vi "UI-RT Communication.vi"(8 "error in (no error)":errorcluster) -> (0 "error out":errorcluster)   [LabVIEW 2016]
uses:
  Controls/Message Structure.ctl
  Controls/Operational Modes.ctl
  Controls/Shutter Manual.ctl
  Controls/Flip Mirror Manual.ctl
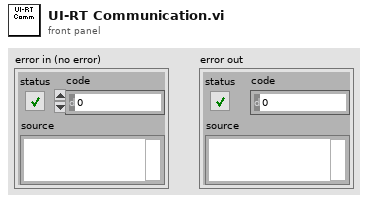
[diagram p1: front panel]
types:
  T1 = typedef "Message Structure.ctl" = cluster{"Data":variant, "Cmd":string}
  T2 = typedef "Operational Modes.ctl" = enum16{"Sci", "Sci-LFC", "Solar", "Solar-LFC", "LFC", "LFC-Sim", "LFC-Both", "ThAr", "ThAr-LFC", "Flat", "ExtFlat", "ExtFlat-Sim", "ExtFlat-Both", "Qtz", "ExtQtz", "ExtQtz-Sim", "ExtQtz-Both", "Dark", "Manual", "Off"}
  T3 = typedef "Shutter Manual.ctl" = cluster{"Science":bool, "Solar":bool, "Ext Flat":bool, "Sim LFC":bool, "Sim Flat":bool}
  T4 = typedef "Flip Mirror Manual.ctl" = cluster{"ExtFlat":bool, "Solar":bool, "ThAr":bool}
  T5 = typedef "Shutters.ctl" = cluster{"Science":T6, "LFCSim":T6, "ExtendFlat":T6, "SimFlat":T6, "Solar":T6}
  T6 = typedef "Shutter Data.ctl" = cluster{"Status":bool, "State":T7, "Time Stamps":cluster{"Open":timestamp, "Close":timestamp}, "Exposure Time":dbl}
  T7 = typedef "Shutter States.ctl" = enum16{"Open", "Close", "Wait", "Off", "Arm", "Idle"}
  T8 = typedef "Flip Mirrors.ctl" = cluster{"ExtFlat":T9, "ThAr":T9, "Solar":T9}
  T9 = typedef "Mirror Data.ctl" = cluster{"Status":bool, "Time Stamp":timestamp}
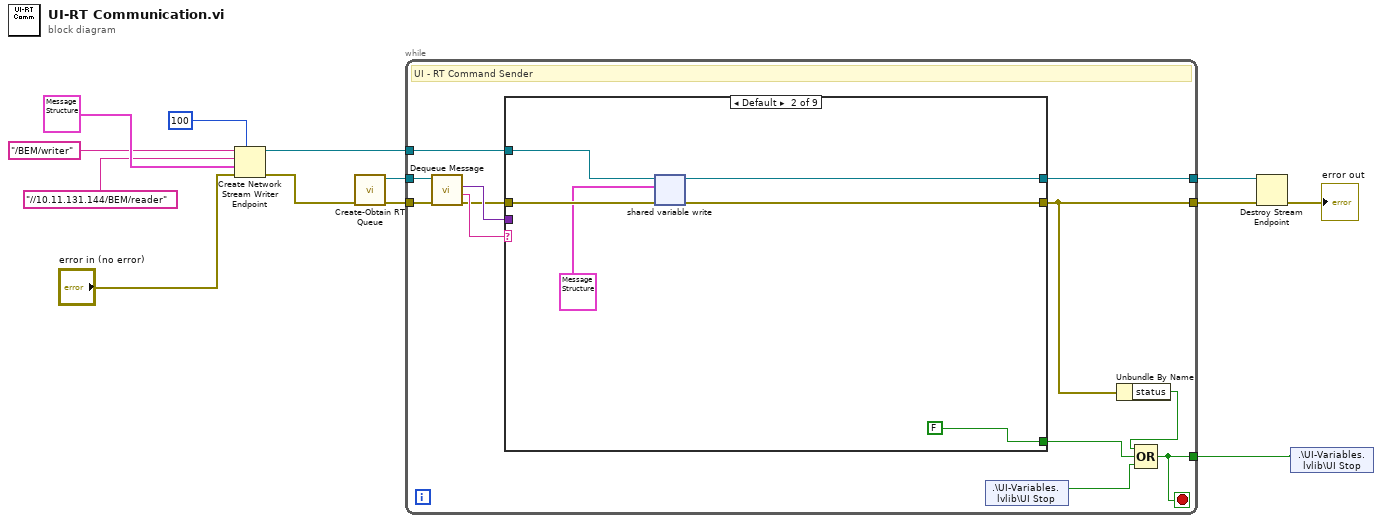
[diagram p0: block diagram]
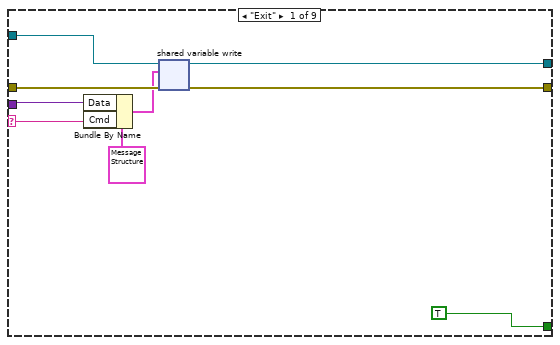
[diagram p2: hidden frame]
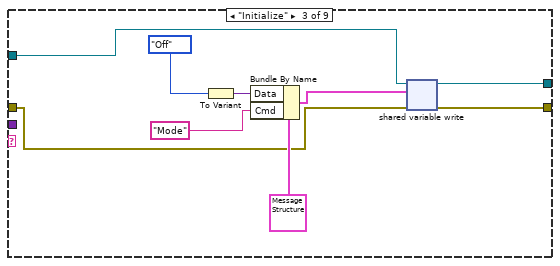
[diagram p3: hidden frame]
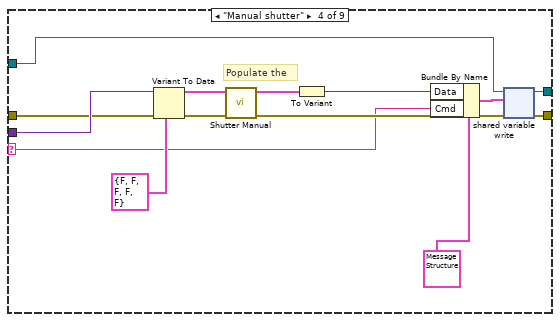
[diagram p4: hidden frame]
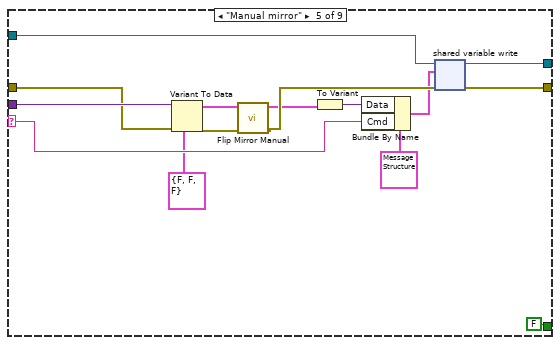
[diagram p5: hidden frame]
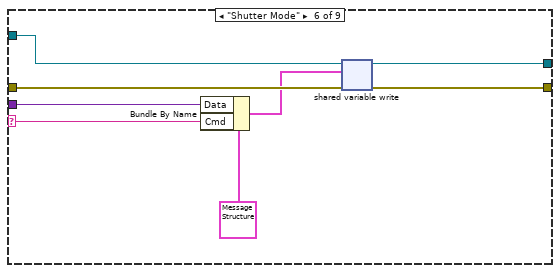
[diagram p6: hidden frame]
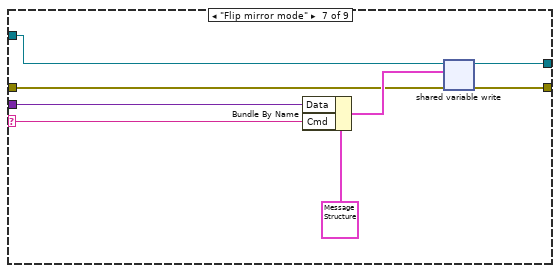
[diagram p7: hidden frame]
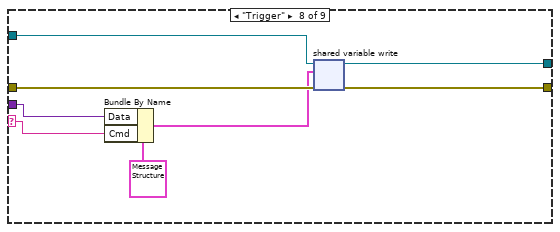
[diagram p8: hidden frame]
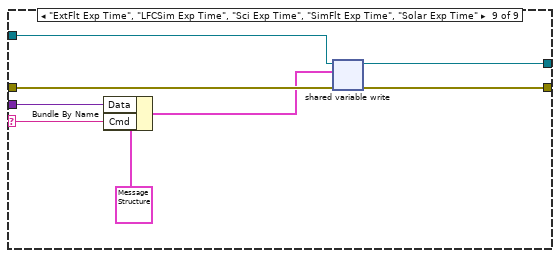
[diagram p9: hidden frame]
diagram:
  n1 = Create Network Stream Writer Endpoint(7:100 ("writer buffer size"), 8:"error in (no error)", 9:T1 {"Data"=variant, "Cmd"=""}, 10:"//10.11.131.144/BEM/reader", 11:"/BEM/writer" ("writer name")) -> (0:w2:errorcluster, 3:w10:refnum<k21>)  [unwired: 2 in]
  n2 = call "Create-Obtain RT Queue.vi"("error in (no error)"=w2) -> ("error out"=w1:errorcluster, "Queue out"=w3:refnum<queue>)  [unwired: 8 in, 1 out]
  n3 = while {
    tunnel: w3 -> [w17]
    tunnel: w10 -> [w25]
    tunnel: [w19] -> w4
    tunnel: w1 -> [w18]
    tunnel: [w22] -> w6
    tunnel: [w21] -> w7
    stop <- w21 stop-if-true
    # "UI - RT Command Sender"
    n4 = call "Dequeue Message.vi"("error in (no error)"=w18, "Queue in"=w17) -> ("error out"=w14:errorcluster, "Cmd"=w16:string, "Data"=w15:variant)  [unwired: 6 in, 1 out]
    n5 = case shown="Default" w16 {
      selector: w16 -> [w27 _ _ w52 w77 w81 w87 w96 w105]
      tunnel: [TRUE FALSE _ _ FALSE _ _ _ _] -> w24
      tunnel: w15 -> [w28 _ _ w63 w76 w82 w88 w97 w104]
      tunnel: w14 -> [w33 w39 w41 w62 w66 w84 w90 w99 w108]
      tunnel: w25 -> [w32 w38 w47 w57 w74 w80 w89 w102 w107]
      tunnel: [w31 w37 w48 w59 w73 w85 w92 w100 w109] -> w19
      tunnel: [w30 w36 w49 w58 w75 w86 w91 w101 w110] -> w22
      frame "Exit" {
        n6 = Bundle By Name(cluster=T1 {"Data"=variant, "Cmd"=""} ("Message"), "Data"=w28, "Cmd"=w27) -> (w26:T1)
        n7 = shared-variable-write(w32, w33, w26) -> (w30:refnum<k21>, w31:errorcluster)  [unwired: 1 in, 1 out]
      }
      frame Default {
        n8 = shared-variable-write(w38, w39, T1 {"Data"=variant, "Cmd"=""} ("Message")) -> (w36:refnum<k21>, w37:errorcluster)  [unwired: 1 in, 1 out]
      }
      frame "Initialize" {
        n9 = To Variant(anything=Operational_Modes."Off" ("EXPRES Mode 2")) -> (Variant=w46:variant)
        n10 = Bundle By Name(cluster=T1 {"Data"=variant, "Cmd"=""} ("Message"), "Data"=w46, "Cmd"="Mode") -> (w43:T1)
        n11 = shared-variable-write(w47, w41, w43) -> (w49:refnum<k21>, w48:errorcluster)  [unwired: 1 in, 1 out]
      }
      frame "Manual shutter" {
        # "Populate the"
        n12 = Variant To Data(error in=w62, type=T3 {"Science"=FALSE, "Solar"=FALSE, "Ext Flat"=FALSE, "Sim LFC"=FALSE, "Sim Flat"=FALSE} ("Manual Shutter 2"), Variant=w63) -> (data=w60:T3, error out=w55:errorcluster)
        n13 = call "Shutter Manual.vi"("Error In"=w55, "Manual Shutter in"=w60) -> ("Error Out"=w54:errorcluster, "Shutters out"=w53:T5)  [unwired: 8 in]
        n14 = To Variant(anything=w53) -> (Variant=w56:variant)
        n15 = Bundle By Name(cluster=T1 {"Data"=variant, "Cmd"=""} ("Message"), "Data"=w56, "Cmd"=w52) -> (w50:T1)
        n16 = shared-variable-write(w57, w54, w50) -> (w58:refnum<k21>, w59:errorcluster)  [unwired: 1 in, 1 out]
      }
      frame "Manual mirror" {
        n17 = Variant To Data(error in=w66, type=T4 {"ExtFlat"=FALSE, "Solar"=FALSE, "ThAr"=FALSE} ("Manual Mirror"), Variant=w76) -> (data=w68:T4, error out=w71:errorcluster)
        n18 = call "Flip Mirror Manual.vi"("error in (no error)"=w71, "Manual Mirror"=w68) -> ("error out"=w70:errorcluster, "Mirrors"=w69:T8)  [unwired: 8 in]
        n19 = To Variant(anything=w69) -> (Variant=w78:variant)
        n20 = Bundle By Name(cluster=T1 {"Data"=variant, "Cmd"=""} ("Message"), "Data"=w78, "Cmd"=w77) -> (w65:T1)
        n21 = shared-variable-write(w74, w70, w65) -> (w75:refnum<k21>, w73:errorcluster)  [unwired: 1 in, 1 out]
      }
      frame "Shutter Mode" {
        n22 = Bundle By Name(cluster=T1 {"Data"=variant, "Cmd"=""} ("Message"), "Data"=w82, "Cmd"=w81) -> (w79:T1)
        n23 = shared-variable-write(w80, w84, w79) -> (w86:refnum<k21>, w85:errorcluster)  [unwired: 1 in, 1 out]
      }
      frame "Flip mirror mode" {
        n24 = Bundle By Name(cluster=T1 {"Data"=variant, "Cmd"=""} ("Message"), "Data"=w88, "Cmd"=w87) -> (w94:T1)
        n25 = shared-variable-write(w89, w90, w94) -> (w91:refnum<k21>, w92:errorcluster)  [unwired: 1 in, 1 out]
      }
      frame "Trigger" {
        n26 = Bundle By Name(cluster=T1 {"Data"=variant, "Cmd"=""} ("Message"), "Data"=w97, "Cmd"=w96) -> (w95:T1)
        n27 = shared-variable-write(w102, w99, w95) -> (w101:refnum<k21>, w100:errorcluster)  [unwired: 1 in, 1 out]
      }
      frame "ExtFlt Exp Time", "LFCSim Exp Time", "Sci Exp Time", "SimFlt Exp Time", "Solar Exp Time" {
        n28 = Bundle By Name(cluster=T1 {"Data"=variant, "Cmd"=""} ("Message"), "Data"=w104, "Cmd"=w105) -> (w103:T1)
        n29 = shared-variable-write(w107, w108, w103) -> (w110:refnum<k21>, w109:errorcluster)  [unwired: 1 in, 1 out]
      }
    }
    n30 = shared-variable ".\\UI-Variables.lvlib\\UI Stop"() -> (w23:bool)  [unwired: 1 in, 1 out]
    n31 = Unbundle By Name(w19) -> ("status"=w20:bool)
    n32 = Compound Arithmetic op=OR(w20, w24, w23) -> (w21:bool)
  }
  n33 = Destroy Stream Endpoint(8:w4, 11:w6) -> (0:→"error out":errorcluster)
  n34 = shared-variable ".\\UI-Variables.lvlib\\UI Stop"(w7) -> ()  [unwired: 1 in, 1 out]
